vi "GetSlaveStatus.vi"() -> ()   [LabVIEW 2015]
uses:
  State.ctl
panel:
  out "Numeric":i32
  out "error out":errorcluster
  in  "update writer strings":bool
  out "data out":T1
  in  "shared variable refnum in":refnum<k21>="ni.var.psp://localhost/MyToolsStatus/status"
  in  "stop":bool
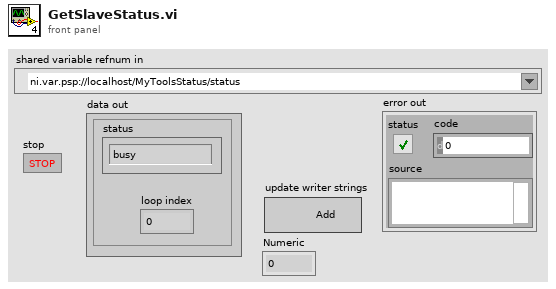
[diagram p1: front panel]
types:
  T1 = typedef "State.ctl" = cluster{"loop index":i32, "status":enum16{"busy", "ready", "error"}}
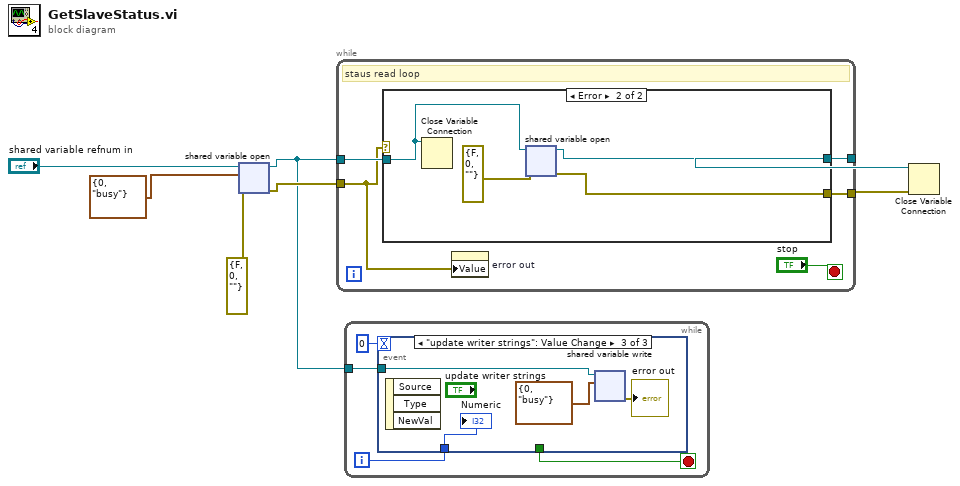
[diagram p0: block diagram]
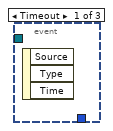
[diagram p2: hidden frame]
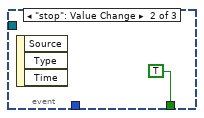
[diagram p3: hidden frame]
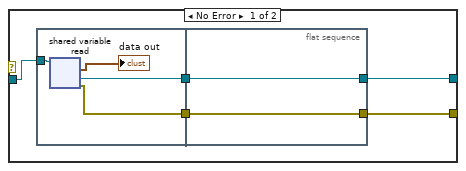
[diagram p4: hidden frame]
diagram:
  n1 = shared-variable-open("shared variable refnum in", errorcluster {"status"=FALSE, "code"=0, "source"=""} ("error in (no error)"), T1 {"loop index"=0, "status"=enum."busy"} ("Enum")) -> (w1:refnum<k21>, w7:errorcluster)  [unwired: 1 in]
  n2 = while {
    tunnel: w1 -> [w11]
    tunnel: w7 -> [w8]
    tunnel: [w10] -> w6
    tunnel: [w9] -> w5
    stop <- "stop" stop-if-true
    # "staus read loop"
    n3 = case shown="Error" w8 {
      tunnel: w11 -> [w17 w25]
      tunnel: [w16 w26] -> w10
      tunnel: [w15 w24] -> w9
      frame No Error {
        n4 = flat-sequence {
          tunnel: w17 -> [w21]
          tunnel: [w20] -> w14
          tunnel: [w19] -> w13
          tunnel: [w22] -> w15
          tunnel: [w23] -> w16
          tunnel: w14 -> [w23]
          tunnel: w13 -> [w22]
          frame #0 {
            n5 = shared-variable-read(w21) -> (w19:refnum<k21>, w20:errorcluster, →"data out":T1)  [unwired: 1 in, 1 out]
          }
          frame #1 {
          }
        }
      }
      frame Error {
        n6 = Close Variable Connection(11:w25) -> ()  [unwired: 1 in, 1 out]
        n7 = shared-variable-open(w25, errorcluster {"status"=FALSE, "code"=0, "source"=""} ("error in (no error)")) -> (w24:refnum<k21>, w26:errorcluster)  [unwired: 1 in]
      }
    }
    n8 = property on="error out" class="Clust (strict)"("Value"=w8) -> ()  [unwired: 2 in, 2 out]
  }
  n9 = while {
    tunnel: w1 -> [w29]
    i -> [w28]
    stop <- w31 stop-if-true
    n10 = event shown="[2] \"update writer strings\": Value Change" {
      selector: _ -> [_ _ _]
      dyn-events: _ -> [_ _ _]
      timeout: 0 -> [_ _ _]
      tunnel: [_ TRUE _] -> w31
      tunnel: w29 -> [_ _ w36]
      tunnel: w28 -> [_ _ w33]
      event Timeout {
        n11 = event-data() -> ()  [unwired: 1 in, 3 out]
      }
      event "stop": Value Change {
        n12 = event-data() -> ()  [unwired: 1 in, 3 out]
      }
      event "update writer strings": Value Change {
        n13 = event-data() -> ()  [unwired: 1 in, 3 out]
        n14 = shared-variable-write(w36, T1 {"loop index"=0, "status"=enum."busy"} ("Enum")) -> (→"error out":errorcluster)  [unwired: 1 in, 1 out]
        "Numeric" <- w33
      }
    }
  }
  n15 = Close Variable Connection(8:w6, 11:w5) -> ()  [unwired: 1 out]
